vi "add return value.vi"(7 "error":bool, 8 "error in (no error)":errorcluster, 10 "JSON Value in":variant, 11 "Cluster in":variant) -> (0 "error out":errorcluster, 3 "Cluster out":variant)   [LabVIEW 2017, in "JSONRPC Server.lvclass"]
uses:
  JSONRPC Server.lvclass
  <vilib>/National Instruments/Variant Data Manipulation/Insert Element at End.vi
  <vilib>/National Instruments/Variant Data Manipulation/Variant Data Manipulation.lvlib
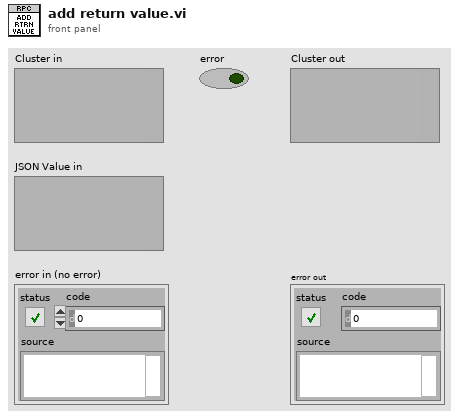
[diagram p1: front panel]
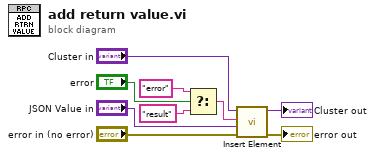
[diagram p0: block diagram]
diagram:
  n1 = Select(t="error", s="error", f="result") -> (s? t:f=w6:string)
  n2 = call-poly <vilib>:"Insert Element.vi"("error in (no error)"="error in (no error)", "element"="JSON Value in", "Name"=w6, "Cluster in"="Cluster in") -> ("error out"=→"error out":errorcluster, "Cluster out"=→"Cluster out":variant)  [unwired: 6 in]
